vi "generate default line.vi"(7 "EthernetIP configuration":refnum<class "EthernetIP configuration.lvclass">, 8 "error in":errorcluster, 11 "operations table":T2) -> (0 "error out":errorcluster, 2 "line":T1)   [LabVIEW 2013, in "EthernetIP editor node.lvclass"]
uses:
  EthernetIP editor node.lvclass
  table reference.ctl
  table line.ctl
  <vilib>/NI/TBM Modules/Ethernet IP/channel/EthernetIP Channel.lvclass
  <vilib>/NI/TBM Modules/Ethernet IP/configuration/EthernetIP configuration.lvclass
  <vilib>/NI/Tag Bus/tag/Data Type.ctl
  <vilib>/NI/TBM Modules/Ethernet IP/configuration/EthernetIP configuration.lvclass/EthernetIP configuration.ctl
  <vilib>/NI/Tag Bus/tag/tag descriptor.lvclass/tag descriptor.ctl
  <vilib>/NI/TBM Modules/Ethernet IP/configuration/Read assemblies.vi
  <vilib>/NI/Tag Bus/tag/tag descriptor.lvclass
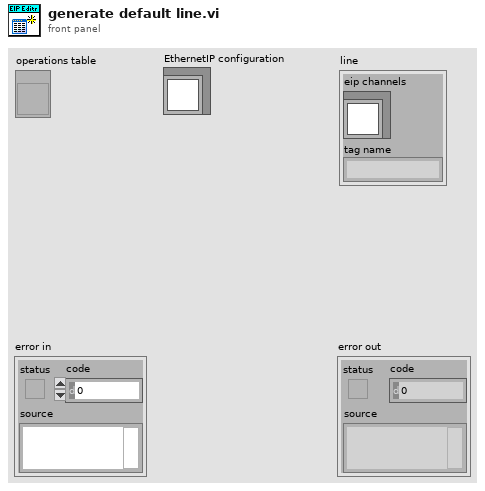
[diagram p1: front panel]
types:
  T1 = typedef "EthernetIP editor node.lvclass/table line.ctl" = cluster{"eip channels":refnum<class "EthernetIP Channel.lvclass">, "tag name":string}
  T2 = typedef "EthernetIP editor node.lvclass/table reference.ctl" = refnum<vi>
  T3 = typedef "tag bus.lvlib/tag descriptor.lvclass/Data Type.ctl" = enum16{"Double", "Single", "I64", "I32", "I16", "I8", "U64", "U32", "U16", "U8", "Boolean", "String", "Array of Double", "Array of Single", "Array of I64", "Array of I32", "Array of I16", "Array of I8", "Array of U64", "Array of U32", "Array of U16", "Array of U8", "Array of Boolean", "Array of String"}
  T4 = typedef "EthernetIP configuration.lvclass/assembly definition.ctl" = cluster{"name":string, "Instance ID":u32, "Type":T5, "Size (bytes)":u32}
  T5 = typedef "EthernetIP configuration.lvclass/assembly type.ctl" = enum32{"Producing", "Consuming"}
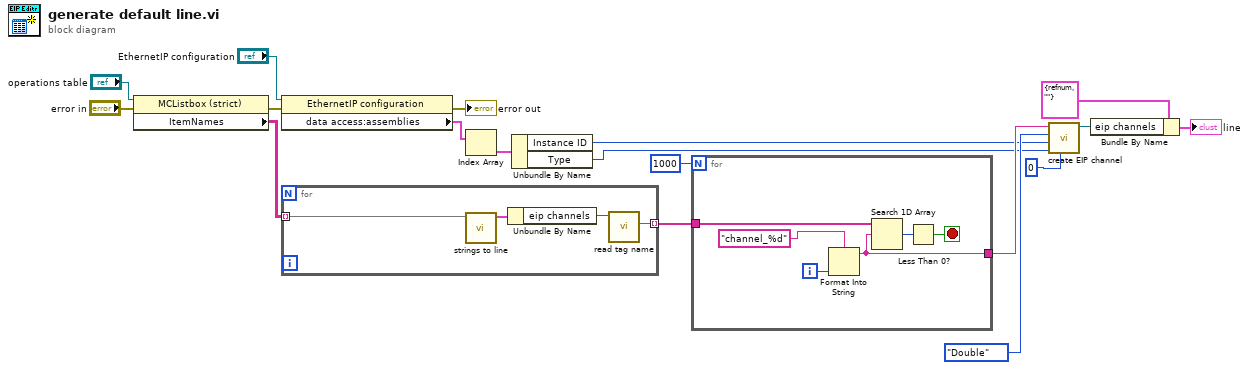
[diagram p0: block diagram]
diagram:
  n1 = property class="MCListbox (strict)"(reference="operations table", error in="error in") -> (error out=w17:errorcluster, "ItemNames"=w15:string[][])  [unwired: 1 out]
  n2 = property class="EthernetIP configuration"(reference="EthernetIP configuration", error in=w17) -> (error out=→"error out":errorcluster, "data access:assemblies"=w4:T4[])  [unwired: 1 out]
  n3 = for {
    tunnel: w15 -> [w22] mode=indexing
    tunnel: [w19] -> w13 mode=indexing
    n4 = call "strings to line.vi"("strings"=w22) -> ("line"=w21:T1)  [unwired: 10 in]
    n5 = Unbundle By Name(w21) -> ("eip channels"=w20:refnum<class "EthernetIP Channel.lvclass">)
    n6 = call <vilib>:"read tag name.vi"("system tag in"=w20) -> ("name"=w19:string)  [unwired: 8 in, 2 out]
  }
  n7 = Index Array(array=w4) -> (element=w3:T4)  [unwired: 1 in]
  n8 = Unbundle By Name(w3) -> ("Instance ID"=w2:u32, "Type"=w1:T5)
  n9 = for {
    N: 1000 -> [_]
    tunnel: w13 -> [w26]
    tunnel: [w23] -> w9
    i -> [w28]
    stop <- w24 stop-if-true
    n10 = Format Into String(format string="channel_%d", w28) -> (resulting string=w23:string)  [unwired: 2 in, 1 out]
    n11 = Search 1D Array(1D array=w26, element=w23) -> (index of element=w25:i32)  [unwired: 1 in]
    n12 = Less Than 0?(x=w25) -> (x < 0?=w24:bool)
  }
  n13 = call <vilib>:"create EIP channel.vi"("byte index"=0, "Type"=w1, "Instance ID"=w2, "data type"=Data_Type."Double", "name"=w9) -> ("EthernetIP Channel out"=w10:refnum<class "EthernetIP Channel.lvclass">)  [unwired: 6 in]
  n14 = Bundle By Name(cluster=T1 {"eip channels"=refnum, "tag name"=""} ("line"), "eip channels"=w10) -> (→"line":T1)
